vi "选择留样瓶对话框.vi"(11 "选择留样瓶":u16) -> (2 "布尔":bool=TRUE, 3 "选择留样瓶 2":u16)   [LabVIEW 2016, in "超标留样集成.lvlib" / "ESTD1200.lvlib"]
uses:
  ESTD1200.lvlib
  <vilib>/Utility/miscctls.llb/LVPointTypeDef.ctl
panel:
  in  "取消":bool
  in  "确定":bool
  # "请选择留样瓶号1~12"
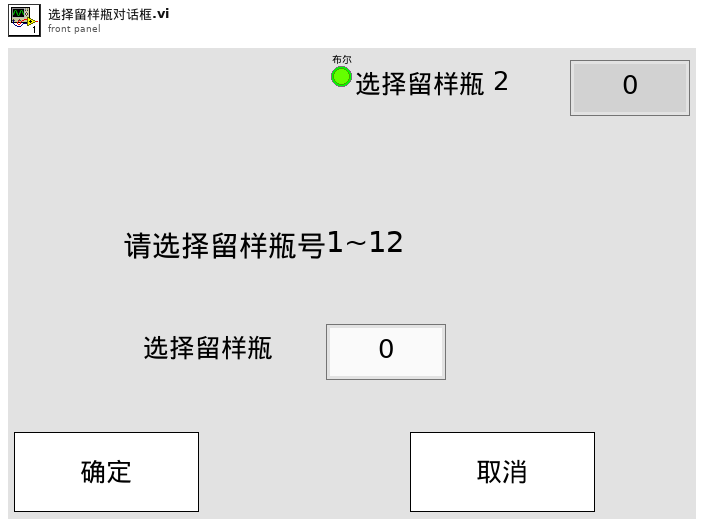
[diagram p1: front panel]
types:
  T1 = typedef "LVPointTypeDef.ctl" = cluster{"Horizontal":i16, "Vertical":i16}
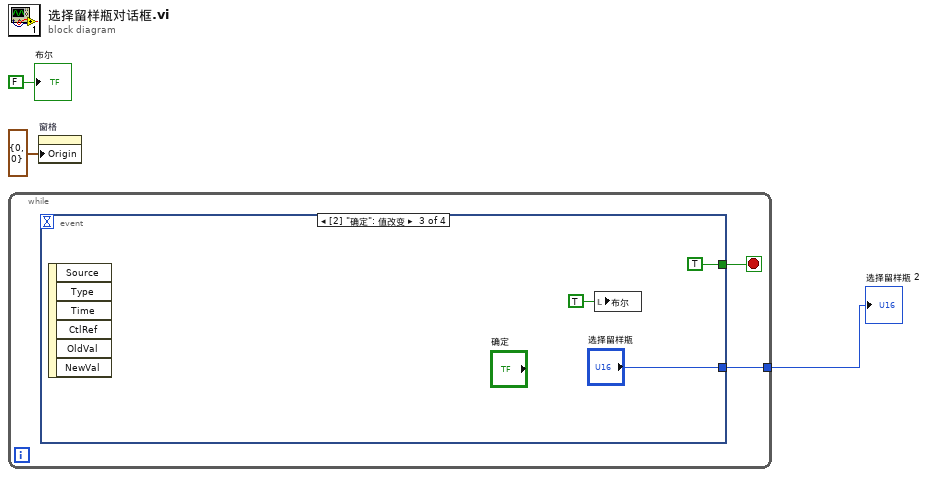
[diagram p0: block diagram]
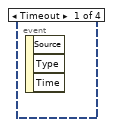
[diagram p2: hidden frame]
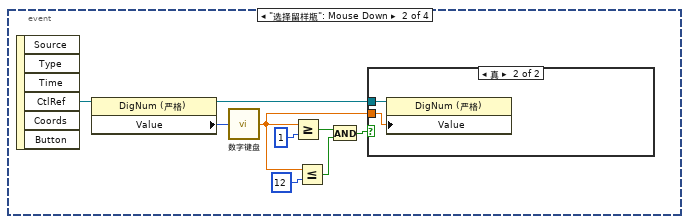
[diagram p3: hidden frame]
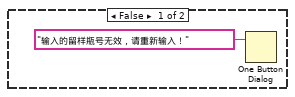
[diagram p4: hidden frame]
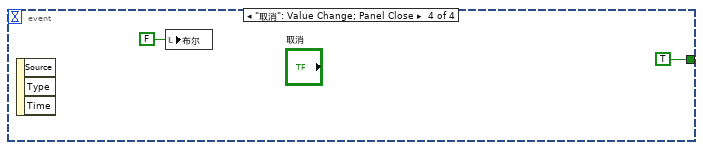
[diagram p5: hidden frame]
diagram:
  n1 = while {
    tunnel: [w4] -> w1
    stop <- w5 stop-if-true
    n2 = event shown="[2] \"确定\": 值改变" {
      selector: _ -> [_ _ _ _]
      dyn-events: _ -> [_ _ _ _]
      timeout: _ -> [_ _ _ _]
      tunnel: [_ _ TRUE TRUE] -> w5
      tunnel: [_ _ "选择留样瓶" _] -> w4
      event Timeout {
        n3 = event-data() -> ()  [unwired: 1 in, 3 out]
      }
      event "选择留样瓶": Mouse Down {
        n4 = event-data() -> ("CtlRef"=w14:refnum<vi>)  [unwired: 1 in, 5 out]
        n5 = property class="DigNum (严格)"(reference=w14) -> (reference out=w13:refnum<vi>, "Value"=w12:u16)  [unwired: 1 in, 1 out]
        n6 = call "数字键盘.vi"("OldNumber"=w12) -> ("NewNumber"=w10:sgl)
        n7 = Greater Or Equal?(x=w10, y=u16 1) -> (x >= y?=w8:bool)
        n8 = Less Or Equal?(x=w10, y=u16 12) -> (x <= y?=w7:bool)
        n9 = And(x=w8, y=w7) -> (x .and. y?=w6:bool)
        n10 = case shown="真" w6 {
          tunnel: w13 -> [_ w17]
          tunnel: w10 -> [_ w16]
          frame False {
            n11 = One Button Dialog(message="输入的留样瓶号无效，请重新输入！" ("消息")) -> ()  [unwired: 1 in, 1 out]
          }
          frame True {
            n12 = property class="DigNum (严格)"(reference=w17, "Value"=w16) -> ()  [unwired: 1 in, 2 out]
          }
        }
      }
      event "确定": Value Change {
        n13 = event-data() -> ()  [unwired: 1 in, 6 out]
        n14 = local write "布尔"(TRUE ("布尔")) -> ()
      }
      event "取消": Value Change; Panel Close {
        n15 = event-data() -> ()  [unwired: 1 in, 3 out]
        n16 = local write "布尔"(FALSE ("布尔")) -> ()
      }
    }
  }
  "选择留样瓶 2" <- w1
  n17 = property on="窗格" class="Pane"("Origin"=T1 {"Horizontal"=0, "Vertical"=0} ("原点")) -> ()  [unwired: 2 in, 2 out]
  "布尔" <- FALSE ("布尔")
